vi "Bar position.vi"(6 "bar width (pix)":dbl, 8 "frequency (Hz)":dbl, 9 "amplitude (pix/s)":dbl, 10 "speed (pix/s)":dbl, 11 "time (s)":dbl) -> (3 "position out":dbl)   [LabVIEW 2012]
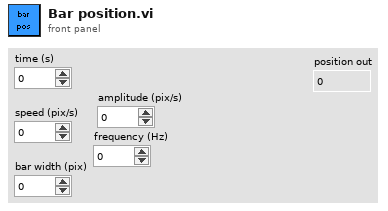
[diagram p1: front panel]
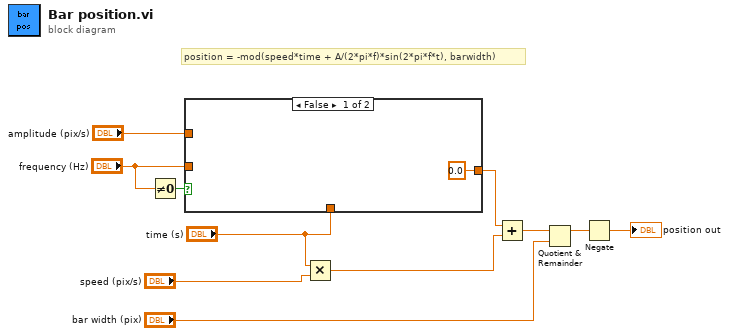
[diagram p0: block diagram]
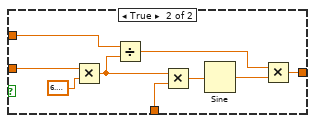
[diagram p2: hidden frame]
diagram:
  # "position = -mod(speed*time + A/(2*pi*f)*sin(2*pi*f*t), barwidth)"
  n1 = Not Equal To 0?(x="frequency (Hz)") -> (x != 0?=w1:bool)
  n2 = case shown="False" w1 {
    tunnel: "frequency (Hz)" -> [_ w21]
    tunnel: "amplitude (pix/s)" -> [_ w19]
    tunnel: "time (s)" -> [_ w17]
    tunnel: [0.0 w13] -> w8
    frame False {
    }
    frame True {
      n3 = Multiply(x=w21, y=6.283185307179586) -> (x*y=w18:dbl)
      n4 = Divide(x=w19, y=w18) -> (x/y=w14:dbl)
      n5 = Multiply(x=w18, y=w17) -> (x*y=w16:dbl)
      n6 = Sine(x=w16) -> (sin(x)=w15:dbl)
      n7 = Multiply(x=w14, y=w15) -> (x*y=w13:dbl)
    }
  }
  n8 = Multiply(x="time (s)", y="speed (pix/s)") -> (x*y=w7:dbl)
  n9 = Add(x=w8, y=w7) -> (x+y=w6:dbl)
  n10 = Quotient & Remainder(x=w6, y="bar width (pix)") -> (x-y*floor(x/y)=w4:dbl)  [unwired: 1 out]
  n11 = Negate(x=w4) -> (-x=→"position out":dbl)
